vi "PD500 - Local Sense Test TSFTS2_v2.vi"(8 "Error In":errorcluster, 10 "Board Selector":T1, 11 "Control Board VISA":refnum<visa-resource-name>) -> (0 "Error Out":errorcluster, 2 "Message OUT":string, 3 "Pass?":bool)   [LabVIEW 2022 SP3]
uses:
  Serial Board Com/Board Select.ctl
panel:
  out "MSE Array":dbl[](array[numeric])
  out "Voltage Readings":dbl[][](array[numeric])
  in  "Message IN":string
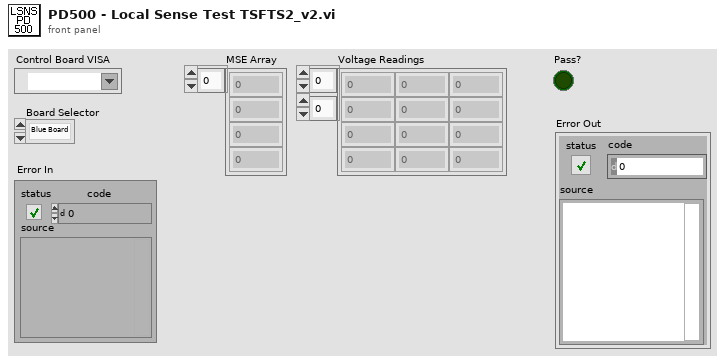
[diagram p1: front panel]
types:
  T1 = typedef "Board Select.ctl" = enum16{"Blue Board", "Green Board"}
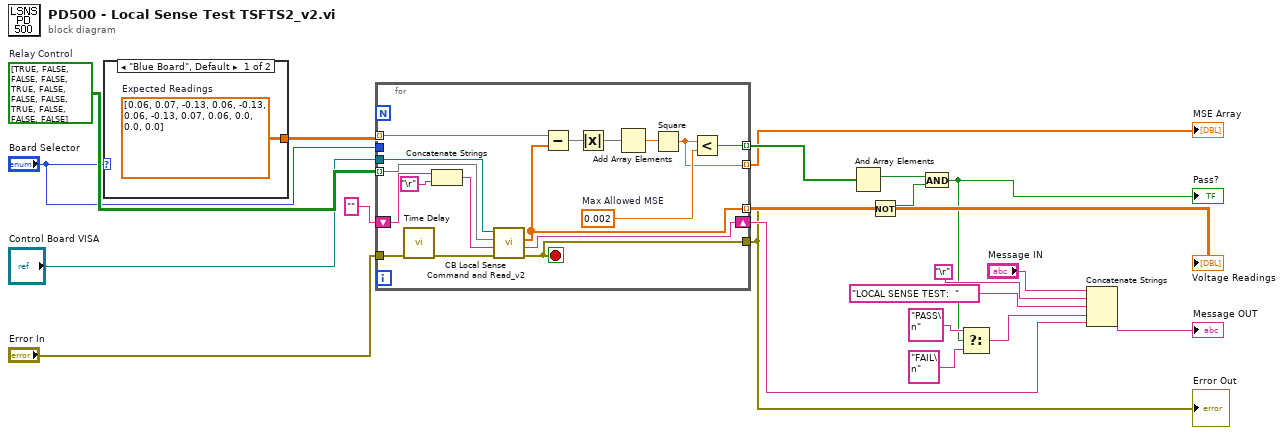
[diagram p0: block diagram]
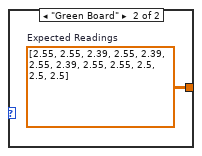
[diagram p2: hidden frame]
diagram:
  w19 = bool[][] [[TRUE, FALSE, FALSE], [FALSE, TRUE, FALSE], [FALSE, FALSE, TRUE], [FALSE, FALSE, FALSE]]  # Relay Control
  n1 = case shown="\"Blue Board\", Default" "Board Selector" {
    tunnel: [w22 w23] -> w21
    frame "Blue Board", Default {
      w22 = dbl[][] [[0.06, 0.07, -0.13], [0.06, -0.13, 0.06], [-0.13, 0.07, 0.06], [0.0, 0.0, 0.0]]  # Expected Readings
    }
    frame "Green Board" {
      w23 = dbl[][] [[2.55, 2.55, 2.39], [2.55, 2.39, 2.55], [2.39, 2.55, 2.55], [2.5, 2.5, 2.5]]  # Expected Readings
    }
  }
  n2 = for {
    tunnel: [w40] -> w2
    tunnel: "Error In" -> [w26]
    tunnel: w21 -> [w37] mode=indexing
    tunnel: [w34] -> w20 mode=indexing
    tunnel: w19 -> [w33] mode=indexing
    tunnel: [w32] -> w16 mode=indexing
    tunnel: [w31] -> w15 mode=indexing
    shift-right: [w30] -> w8
    shift-left: "" -> [w29]
    tunnel: "Board Selector" -> [_]
    tunnel: "Control Board VISA" -> [w24]
    stop <- w40 stop-if-true
    w35 = 0.002  # Max Allowed MSE
    n3 = call "Time Delay"("error in (no error)"=w26) -> ("error out"=w25:errorcluster)  [unwired: 10 in]
    n4 = Concatenate Strings(w29, "\r") -> (w28:string)
    n5 = call "CB Local Sense Command and Read_v2.vi"("error in (no error)"=w25, "Message IN"=w28, "Relay Control"=w33, "Control Board VISA"=w24) -> ("error out"=w40:errorcluster, "Message OUT"=w30:string, "Voltage Array"=w32:dbl[])  [unwired: 4 in, 1 out]
    n6 = Subtract(x=w37, y=w32) -> (x-y=w39:dbl[])
    n7 = Absolute Value(x=w39) -> (abs(x)=w38:dbl[])
    n8 = Add Array Elements(numeric array=w38) -> (sum=w36:dbl)
    n9 = Square(x=w36) -> (x^2=w31:dbl)
    n10 = Less?(x=w31, y=w35) -> (x < y?=w34:bool)
  }
  "Voltage Readings" <- w16
  "MSE Array" <- w15
  "Error Out" <- w2
  n11 = And Array Elements(Boolean array=w20) -> (logical AND=w18:bool)
  n12 = Not(x=w2) -> (.not. x?=w17:bool)
  n13 = And(x=w18, y=w17) -> (x .and. y?=w10:bool)
  "Pass?" <- w10
  n14 = Select(t="PASS\n", s=w10, f="FAIL\n") -> (s? t:f=w9:string)
  n15 = Concatenate Strings("Message IN", "\r", "LOCAL SENSE TEST:  ", w9, w8) -> (→"Message OUT":string)
